vi "Dashboard Main.vi"() -> ()   [LabVIEW 2013]
uses:
  <vilib>/event_ctls.llb/eventvkey.ctl
  <vilib>/Rock Robotics/WPI/Dashboard/WPI_DashboardLogging Global.vi
  <vilib>/Utility/config.llb/Write Key (String).vi
  <vilib>/Utility/config.llb/Write Key (I32).vi
  <vilib>/Utility/config.llb/NI_LVConfig.lvlib
panel:
  out "Image Message":string="Timeout in Camera Communications"
  in  "Rec Mode":enum32{"Stop", "Record", "Playback"}(radio)
  in  "Dashboard Tab":T1(tab)
  out "Meter":dbl(knob) caption="Catapult Pressure" scale=0.0..100.0
  out "TapeMeasure":dbl caption="Distance To Target" format="%#_4g"
  out "CatapultLocked":bool caption="Catapult"
  out "TRghtStop":bool caption="Turret Right Stop"
  out "TLftStop":bool caption="Turret Left Stop"
  in  "Camera Settings":T2={"Frame Rate"=30, "Compression"=30, "Size"=1} {"Frame Rate" scale=1.0..30.0; "Size" items=["640x480", "320x240", "160x120"]}
  out "MotorSliders R":cluster{"MotorSlide1":dbl, "MotorSlide2":dbl} {"MotorSlide2" scale=-1.0..1.0 scale format="%#_2e"; "MotorSlide1" scale=-1.0..1.0 scale format="%#_2e"}
  out "MotorChart R":cluster{"Numeric":dbl, "Numeric":dbl}(graph)
  out "MotorSliders L":T3 {"MotorSlide4 2" scale=0.0..14.0 scale format="%#_2e"; "MotorSlide2" scale=-1.0..1.0 scale format="%#_2e"; "MotorSlide1" scale=-1.0..1.0 scale format="%#_2e"}
  out "MotorChart L":T4(graph)
  out "JS1 Z":dbl(slide) scale=-1.0..1.0 scale format="%#_2e"
  out "Joystick 1":cluster{"X":dbl, "Y":dbl}[](graph)
  out "JS Buttons 1":T5
  out "JS2 Z":dbl(slide) scale=-1.0..1.0 scale format="%#_2e"
  out "Joystick 2":cluster{"X":dbl, "Y":dbl}[](graph)
  out "JS Buttons 2":T5
  out "Mode":T6(ring)=enum."Auto Disabled"
  out "Camera IP":string
  in  "DB Camera Config":bool
  out "fps":dbl format="%#.1g"
  out "Mbps":dbl format="%#.1g"
  out "Mbps 2":bool
  out "JS3 Z":dbl(slide) scale=1.0..-1.0 scale format="%#_2e"
  out "Joystick 3":cluster{"X":dbl, "Y":dbl}[](graph) caption="XBOX"
  out "JS Buttons 3":T5
  in  "Slider 1":dbl(slide) scale=0.0..100.0
  in  "Checkbox 2":bool
  in  "Checkbox 1":bool
  in  "Test Slider":dbl(slide) scale=0.0..100.0 scale format="%#_3g"
  in  "On/Off":bool caption="Solenoid"
  in  "Test Name":u16(ring) items=["Select the test to run...", "Example Test", "-------------------------------", "List of tests is built in robot code.", "Replace with your own automated tests."]
  in  "Test Tree":string(tree)
  in  "Motor":cluster{"Value":dbl, "Enable":bool} {"Value" scale=-1.0..1.0 scale format="%#_3g"}
  out "Progress":T7 {"Test Progress" scale=0.0..100.0}
  in  "Rev/Fwd":cluster{"Forward":bool, "Reverse":bool}
  in  "Test Ring":u16(ring) items=["Auto", "Fixed indoor", "Fixed outdoor 1", "Fixed outdoor 2", "Fixed fluorescent 1", "Fixed fluorescent 2", "Hold current"]
  in  "Listbox":i32(listbox)
  out "Tree":string(tree)
  out "Camera Image":T8(plugin-control)
  in  "Enable":bool
  # "Left"
  # "Front"
  # "Right"
  # "Battery"
  # "Customize by placing controls and indicators here and name to\nmatch Dashboard Variables on robot."
  # "This tab is a great place for autonomous settings and validation.\nCustomize by placing controls and indicators here and name to\nmatch Dashboard Variables on robot."
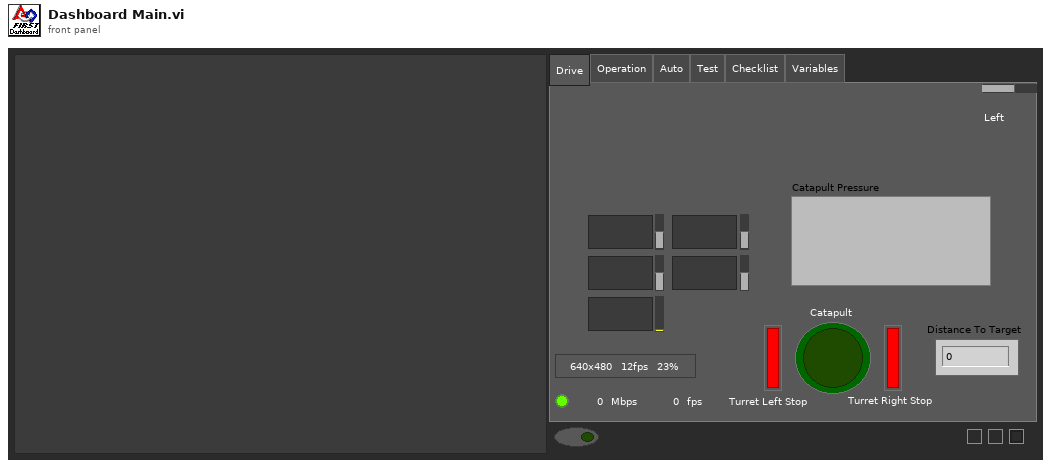
[diagram p1: front panel]
types:
  T1 = enum32{"Drive", "Operation", "Auto", "Test", "Checklist", "Variables"}
  T2 = cluster{"Frame Rate":i32, "Compression":i32, "Size":u16}
  T3 = cluster{"MotorSlide1":dbl, "MotorSlide2":dbl, "MotorSlide4 2":dbl}
  T4 = cluster{"Numeric":dbl, "Numeric":dbl, "Battery":sgl}
  T5 = cluster{bool, bool, bool, bool, bool, bool, bool, bool, bool, bool, bool, bool}
  T6 = enum8{"Tele-Op Disabled", "Tele-Op Enabled", "Auto Disabled", "Auto Enabled", "Test Disabled", "Test Enabled", ""}
  T7 = cluster{"Test Progress":u8, "Test Progress Text":string}
  T8 = typedef "IMAQ Image.ctl" = refnum<image>
  T9 = typedef "Image Type" = u32
  T10 = cluster{"Digital Inputs":bool[], "Digital Outputs":bool[]}
  T11 = cluster{"Competition mode":bool, "Robot Link":bool, "Autonomous":bool, "Enabled":bool, "E-Stop":bool, "Simulated":bool, "TestMode":bool, "Docked Window":bool}
  T12 = cluster{"Boolean Array[0]":bool, "Boolean Array[1]":bool, "Boolean Array[2]":bool, "Boolean Array[3]":bool, "Boolean Array[4]":bool, "Boolean Array[5]":bool, "Boolean Array[6]":bool, "Boolean Array[7]":bool, "Boolean Array[8]":bool, "Boolean Array[9]":bool, "Boolean Array[10]":bool, "Boolean Array[11]":bool}
  T13 = typedef "NI_LVConfig.lvlib/Config Data RefNum.ctl" = refnum<k1>
  T14 = typedef "eventvkey.ctl" = enum16{"ASCII", "Enter", "Return", "Shift", "Ctrl", "Alt", "Cmd", "Opt", "Caps", "NumLock", "Clear", "Break", "Up", "Down", "Left", "Right", "Insert", "Delete", "Home", "End", "PageUp", "PageDown", "Escape", "Help", "Pause", "ScrollLock", "F1", "F2", "F3", "F4", "F5", "F6", "F7", "F8", "F9", "F10", "F11", "F12", "F13", "F14", "F15", "F16", "F17", "F18", "F19", "F20", "F21", "F22", "F23", "F24", "Play", "VolumeUp", "VolumeDown", "Mute", "Two Byte Char"}
  T15 = cluster{"Image Size":bool, "Image Type":bool, "Pixel Value":bool, "ROI Information":bool, "Zoom Factor":bool}
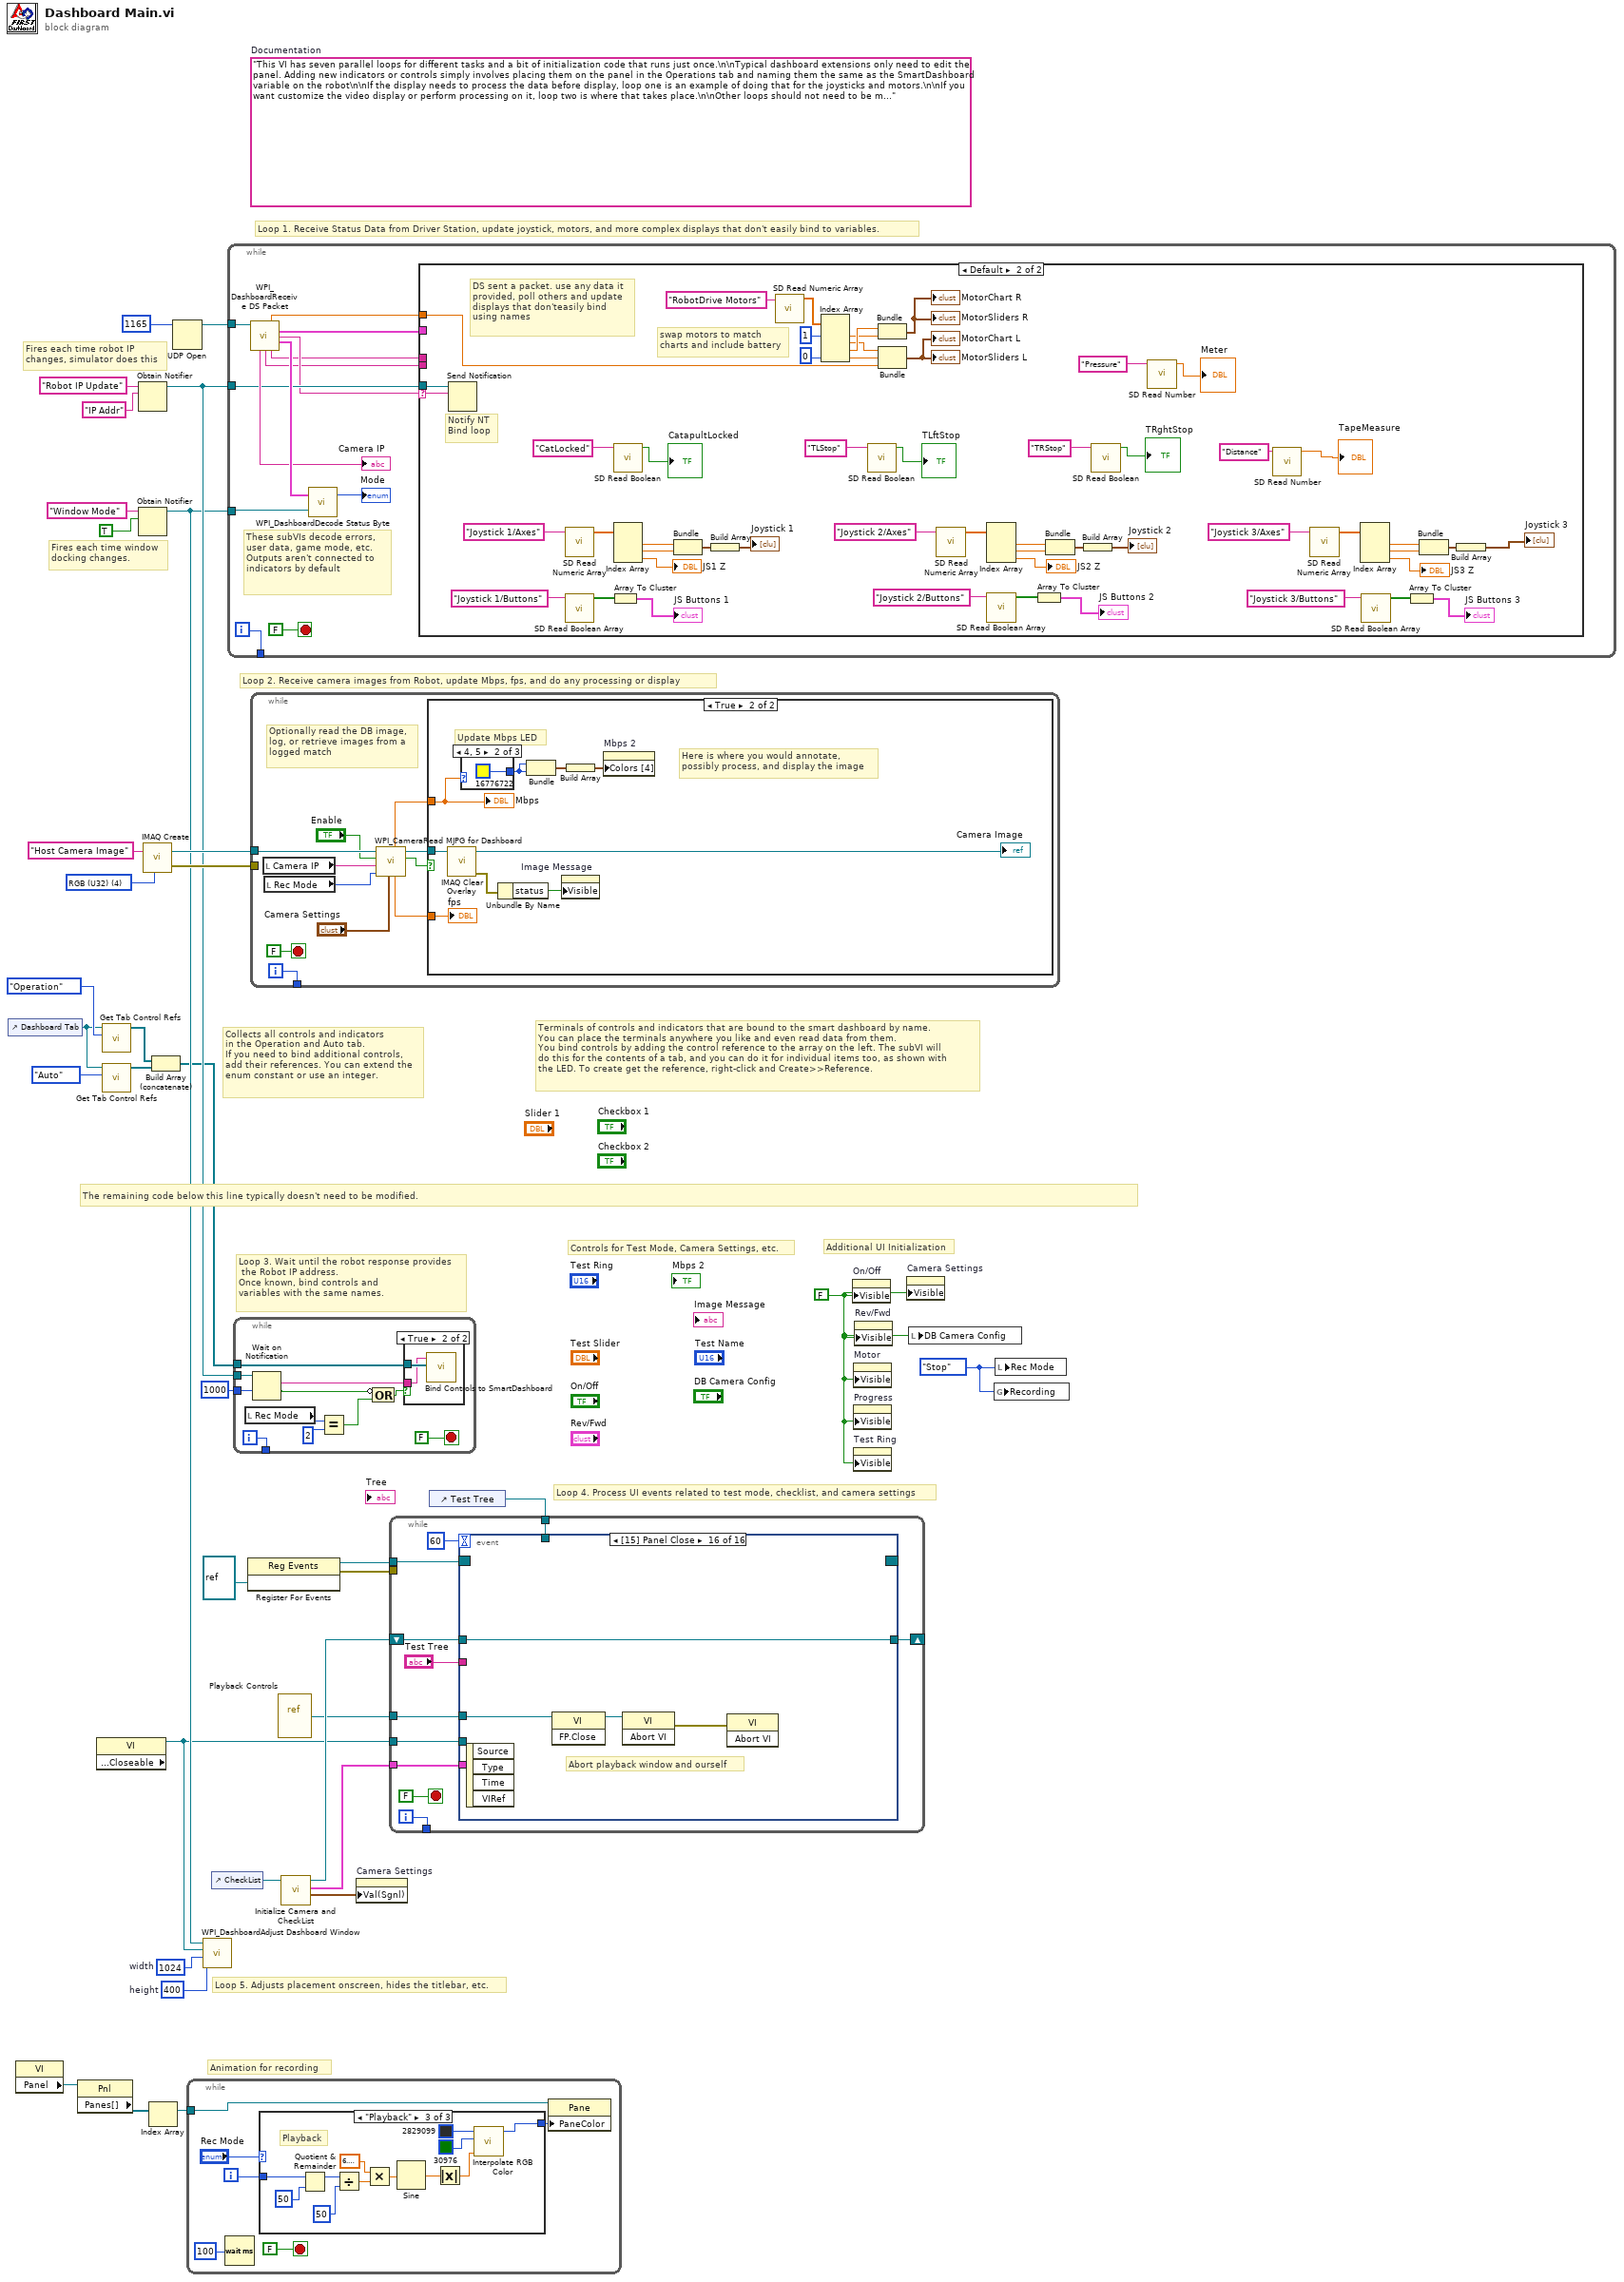
[diagram p0: block diagram]
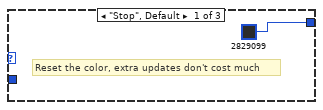
[diagram p2: hidden frame]
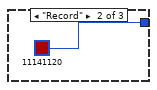
[diagram p3: hidden frame]
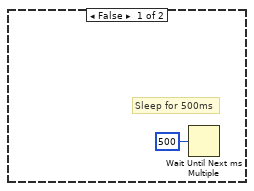
[diagram p5: hidden frame]
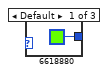
[diagram p6: hidden frame]
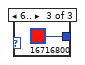
[diagram p7: hidden frame]
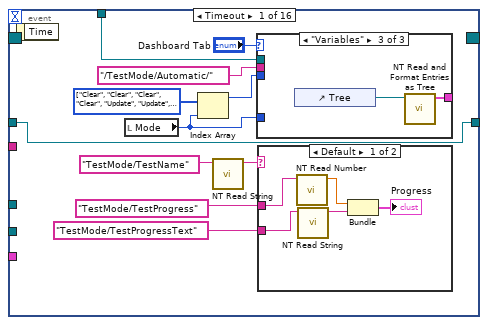
[diagram p8: hidden frame]
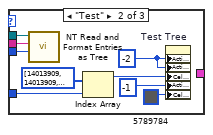
[diagram p10: hidden frame]
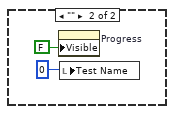
[diagram p11: hidden frame]
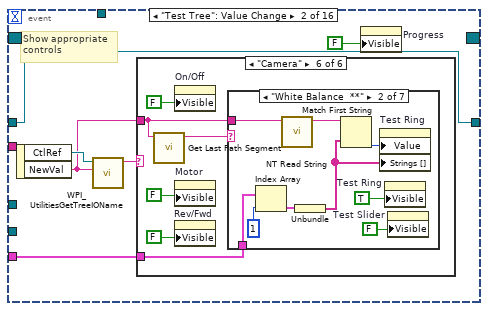
[diagram p12: hidden frame]
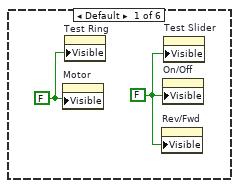
[diagram p13: hidden frame]
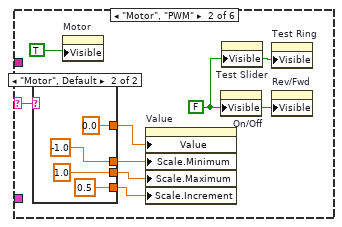
[diagram p14: hidden frame]
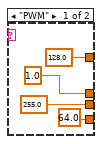
[diagram p15: hidden frame]
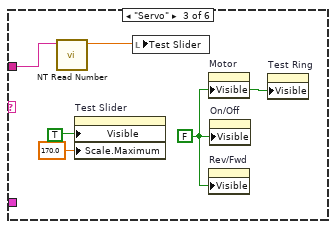
[diagram p16: hidden frame]
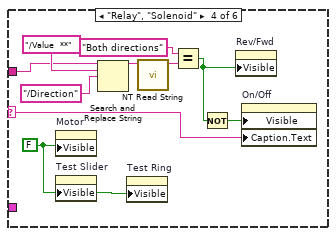
[diagram p17: hidden frame]
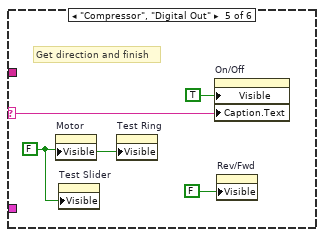
[diagram p18: hidden frame]
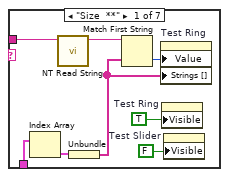
[diagram p19: hidden frame]
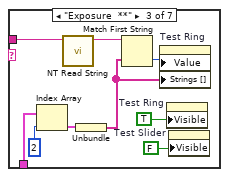
[diagram p20: hidden frame]
diagram:
  w7 = enum32{"Stop", "Record", "Playback"}."Stop" ("Rec Mode")
  w10 = 400  # height
  w11 = 1024  # width
  w24 = FALSE ("Visible")
  (unwired) "This VI has seven parallel loops for different tasks and a bit of initialization code that runs just once.\n\nTypical dashboard extensions only need to edit the panel. Adding new indicators or controls simply involves placing them on the panel in the Operations tab and naming them the same as the SmartDashboard variable on the robot\n\nIf the display needs to process the data before display, loop one is an example of doing that for the joysticks and motors.\n\nIf you want customize the video display or perform processing on it, loop two is where that takes place.\n\nOther loops should not need to be modified. They are pretty standard, and document the task they perform."  # Documentation
  w34 = T9 4 items=["Grayscale (U8)", "Grayscale (I16)", "Grayscale (SGL)", "Complex (CSG)", "RGB (U32)", "HSL (U32)", "RGB (U64)"] ("Image Type")
  # "Controls for Test Mode, Camera Settings, etc."
  # "Additional UI Initialization"
  # "Animation for recording"
  # "Fires each time robot IP\nchanges, simulator does this"
  # "Fires each time window\ndocking changes."
  # "Collects all controls and indicators\nin the Operation and Auto tab.\nIf you need to bind additional controls,\nadd their references. You can extend the\nenum constant or use an integer."
  # "The remaining code below this line typically doesn't need to be modified."
  # "Loop 4. Process UI events related to test mode, checklist, and camera settings"
  # "Terminals of controls and indicators that are bound to the smart dashboard by name.\nYou can place the terminals anywhere you like and even read data from them.\nYou bind controls by adding the control reference to the array on the left. The subVI will\ndo this for the contents of a tab, and you can do it for individual items too, as shown with\nthe LED. To create get the reference, right-click and Create>>Reference."
  # "Loop 3. Wait until the robot response provides\n the Robot IP address.\nOnce known, bind controls and\nvariables with the same names."
  # "Loop 5. Adjusts placement onscreen, hides the titlebar, etc."
  # "Loop 1. Receive Status Data from Driver Station, update joystick, motors, and more complex displays that don't easily bind to variables."
  # "Loop 2. Receive camera images from Robot, update Mbps, fps, and do any processing or display"
  n1 = control-ref of="Dashboard Tab"() -> (w5:refnum<vi>)
  n2 = property class="VI"() -> ("Panel"=w18:refnum<vi>)  [unwired: 2 in, 2 out]
  n3 = property class="Pnl"(reference=w18) -> ("Panes[]"=w19:refnum<vi>[])  [unwired: 1 in, 2 out]
  n4 = property class="VI" props=["Front Panel.Closeable"]() -> (reference out=w6:refnum<vi>)  [unwired: 2 in, 2 out]
  n5 = call <vilib>:"Get Tab Control Refs.vi"("Page Index"=T1."Operation" ("Dashboard Tab"), "TabControl in"=w5) -> ("ControlsOnPage"=w3:refnum<vi>[])  [unwired: 9 in]
  n6 = call <vilib>:"Get Tab Control Refs.vi"("Page Index"=T1."Auto" ("Dashboard Tab"), "TabControl in"=w5) -> ("ControlsOnPage"=w4:refnum<vi>[])  [unwired: 9 in]
  n7 = Obtain Notifier(name (unnamed)="Robot IP Update", notification data type="IP Addr" ("name (unnamed)")) -> (notifier out=w28:refnum<notifier>)  [unwired: 2 in, 2 out]
  n8 = Obtain Notifier(name (unnamed)="Window Mode", notification data type=TRUE) -> (notifier out=w9:refnum<notifier>)  [unwired: 2 in, 2 out]
  n9 = call "IMAQ Create"("Image Name"="Host Camera Image", "Image Type"=w34) -> ("New Image"=w32:T8, "error out"=w31:errorcluster)  [unwired: 2 in, 1 out]
  n10 = Index Array(array=w19) -> (element=w17:refnum<vi>)  [unwired: 1 in]
  n11 = Build Array (concatenate)(w3, w4) -> (w2:refnum<vi>[])
  n12 = UDP Open(11:u16 1165 ("port")) -> (port=w35:refnum<k16>)  [unwired: 2 in, 4 out]
  n13 = while {
    tunnel: w17 -> [w38]
    i -> [w41]
    stop <- FALSE stop-if-true
    n14 = Wait (ms)(milliseconds to wait=u32 100) -> ()  [unwired: 1 out]
    n15 = case shown="\"Playback\"" "Rec Mode" {
      tunnel: w41 -> [_ _ w56]
      tunnel: [u32 2829099 ("Base Color") u32 11141120 ("Target Color") w45] -> w37
      frame "Stop", Default {
        # "Reset the color, extra updates don't cost much"
      }
      frame "Record" {
      }
      frame "Playback" {
        # "Playback"
        n16 = Quotient & Remainder(x=w56, y=u32 50 ("milliseconds to wait")) -> (x-y*floor(x/y)=w52:u32)  [unwired: 1 out]
        n17 = Divide(x=w52, y=u32 50 ("milliseconds to wait")) -> (x/y=w49:dbl)
        n18 = Multiply(x=6.283185307179586, y=w49) -> (x*y=w54:dbl)
        n19 = Sine(x=w54) -> (sin(x)=w53:dbl)
        n20 = Absolute Value(x=w53) -> (abs(x)=w46:dbl)
        n21 = call "Interpolate RGB Color.vi"("Proportion"=w46, "Target Color"=u32 30976, "Base Color"=u32 2829099) -> ("Result Color"=w45:u32)  [unwired: 8 in]
      }
    }
    n22 = property class="Pane"(reference=w38, "PaneColor"=w37) -> ()  [unwired: 1 in, 2 out]
  }
  n23 = call <vilib>:"WPI_DashboardAdjust Dashboard Window.vi"("height"=w10, "width"=w11, "reference in"=w6, "Notifier in"=w9) -> ()  [unwired: 8 in]
  n24 = control-ref of="CheckList"() -> (w8:refnum<vi>)
  n25 = while {
    tunnel: w35 -> [w67]
    tunnel: w28 -> [w62]
    tunnel: w9 -> [w66]
    tunnel: [w63] -> _
    i -> [w63]
    stop <- FALSE stop-if-true
    # "These subVIs decode errors, user data, game mode, etc.\nOutputs aren't connected to indicators by default"
    n26 = call <vilib>:"WPI_DashboardReceive DS Packet.vi"("Recv Socket"=w67) -> ("Battery"=w57:sgl, "Driver Station"=w58:T10, "Robot IP Address"=w61:string, "Status"=w68:T11, "Camera IP Address"=→"Camera IP":string, "Low Priority User Data"=w60:string, "High Priority User Data"=w59:string)  [unwired: 1 in, 7 out]
    n27 = call <vilib>:"WPI_DashboardDecode Status Byte.vi"("Window Mode Notifier"=w66, "Status"=w68) -> ("Mode"=→"Mode":T6)  [unwired: 1 out]
    n28 = case shown="Default" w61 {
      selector: w61 -> [_ w100]
      tunnel: w62 -> [_ w101]
      tunnel: w60 -> [_ _]
      tunnel: w59 -> [_ _]
      tunnel: w58 -> [_ _]
      tunnel: w57 -> [_ w99]
      frame "0.0.0.0" {
        # "DS not sending packets, or no robot exists yet.\nDon't poll the variables"
      }
      frame Default {
        # "Notify NT\nBind loop"
        # "DS sent a packet. use any data it\nprovided, poll others and update\ndisplays that don'teasily bind\nusing names"
        # "swap motors to match\ncharts and include battery"
        n29 = Send Notification(notification=w100, notifier=w101) -> ()  [unwired: 1 in, 2 out]
        n30 = call <vilib>:"SD Read Numeric Array.vi"("Name"="Joystick 1/Axes") -> ("Numeric Array"=w117:dbl[])  [unwired: 8 in, 2 out]
        n31 = call <vilib>:"SD Read Boolean Array.vi"("Name"="Joystick 1/Buttons") -> ("Boolean Array"=w119:bool[])  [unwired: 8 in, 2 out]
        n32 = Array To Cluster(array=w119) -> (cluster=→"JS Buttons 1":T12)
        n33 = call <vilib>:"SD Read Boolean.vi"("Name"="CatLocked") -> ("Boolean"=→"CatapultLocked":bool)  [unwired: 8 in, 2 out]
        n34 = Index Array(array=w117) -> (element #1=w114:dbl, element #2=w115:dbl, element #3=→"JS1 Z":dbl)  [unwired: 3 in]
        n35 = Bundle("Numeric"=w114, "Numeric"=w115) -> (w113:cluster{"Numeric":dbl, "Numeric":dbl})  [unwired: 1 in]
        n36 = Build Array(w113) -> (→"Joystick 1":cluster{"Numeric":dbl, "Numeric":dbl}[])
        n37 = call <vilib>:"SD Read Numeric Array.vi"("Name"="RobotDrive Motors") -> ("Numeric Array"=w98:dbl[])  [unwired: 8 in, 2 out]
        n38 = Index Array(array=w98, index #1=1, index #4=0) -> (element #1=w94:dbl, element #2=w93:dbl, element #3=w95:dbl, element #4=w90:dbl)  [unwired: 2 in]
        n39 = call <vilib>:"SD Read Boolean.vi"("Name"="TLStop") -> ("Boolean"=→"TLftStop":bool)  [unwired: 8 in, 2 out]
        n40 = Bundle("Numeric"=w95, "Numeric"=w94) -> (→"MotorChart R" →"MotorSliders R":cluster{"Numeric":dbl, "Numeric":dbl})  [unwired: 1 in]
        n41 = Bundle("Numeric"=w93, "Numeric"=w90, "Battery"=w99) -> (→"MotorChart L" →"MotorSliders L":T4)  [unwired: 1 in]
        n42 = call <vilib>:"SD Read Numeric Array.vi"("Name"="Joystick 2/Axes") -> ("Numeric Array"=w111:dbl[])  [unwired: 8 in, 2 out]
        n43 = Index Array(array=w111) -> (element #1=w106:dbl, element #2=w105:dbl, element #3=→"JS2 Z":dbl)  [unwired: 3 in]
        n44 = call <vilib>:"SD Read Boolean Array.vi"("Name"="Joystick 2/Buttons") -> ("Boolean Array"=w110:bool[])  [unwired: 8 in, 2 out]
        n45 = Array To Cluster(array=w110) -> (cluster=→"JS Buttons 2":T12)
        n46 = Bundle("Numeric"=w106, "Numeric"=w105) -> (w107:cluster{"Numeric":dbl, "Numeric":dbl})  [unwired: 1 in]
        n47 = Build Array(w107) -> (→"Joystick 2":cluster{"Numeric":dbl, "Numeric":dbl}[])
        n48 = call <vilib>:"SD Read Boolean.vi"("Name"="TRStop") -> ("Boolean"=→"TRghtStop":bool)  [unwired: 8 in, 2 out]
        n49 = call <vilib>:"SD Read Number.vi"("Name"="Pressure") -> ("Numeric"=→"Meter":dbl)  [unwired: 8 in, 2 out]
        n50 = call <vilib>:"SD Read Number.vi"("Name"="Distance") -> ("Numeric"=→"TapeMeasure":dbl)  [unwired: 8 in, 2 out]
        n51 = call <vilib>:"SD Read Numeric Array.vi"("Name"="Joystick 3/Axes") -> ("Numeric Array"=w80:dbl[])  [unwired: 8 in, 2 out]
        n52 = Index Array(array=w80) -> (element #1=w77:dbl, element #2=w76:dbl, element #3=→"JS3 Z":dbl)  [unwired: 3 in]
        n53 = call <vilib>:"SD Read Boolean Array.vi"("Name"="Joystick 3/Buttons") -> ("Boolean Array"=w83:bool[])  [unwired: 8 in, 2 out]
        n54 = Array To Cluster(array=w83) -> (cluster=→"JS Buttons 3":T12)
        n55 = Bundle("Numeric"=w77, "Numeric"=w76) -> (w78:cluster{"Numeric":dbl, "Numeric":dbl})  [unwired: 1 in]
        n56 = Build Array(w78) -> (→"Joystick 3":cluster{"Numeric":dbl, "Numeric":dbl}[])
      }
    }
  }
  n57 = while {
    tunnel: w2 -> [w133]
    tunnel: w28 -> [w131]
    tunnel: [w129] -> _
    tunnel: u32 1000 ("milliseconds to wait") -> [w128]
    i -> [w129]
    stop <- FALSE stop-if-true
    n58 = local read "Rec Mode"() -> (w124:enum32{"Stop", "Record", "Playback"})
    n59 = Wait on Notification(notifier=w131, timeout in ms (-1)=w128) -> (notification=w130:string, timed out?=w126:bool)  [unwired: 2 in, 2 out]
    n60 = Equal?(x=w124, y=u16 2 ("Rec Mode")) -> (x = y?=w125:bool)
    n61 = Compound Arithmetic op=OR(invert w126, w125) -> (w127:bool)
    n62 = case shown="True" w127 {
      tunnel: w133 -> [_ w135]
      tunnel: w130 -> [_ w134]
      frame False {
      }
      frame True {
        n63 = call <vilib>:"Bind Controls to SmartDashboard.vi"("Bound Control Refs"=w135, "Server IP Address"=w134) -> ()  [unwired: 10 in]
      }
    }
  }
  n64 = register-events(refnum<vi> refnum) -> (reference out=w15:refnum<event-registration>, error out=w14:errorcluster)  [unwired: 2 in]
  n65 = while {
    tunnel: w32 -> [w144]
    tunnel: w31 -> [_]
    tunnel: [w145] -> _
    i -> [w145]
    stop <- FALSE stop-if-true
    # "Optionally read the DB image,\nlog, or retrieve images from a\nlogged match"
    n66 = local read "Camera IP"() -> (w137:string)
    n67 = local read "Rec Mode"() -> (w136:enum32{"Stop", "Record", "Playback"})
    n68 = call <vilib>:"WPI_CameraRead MJPG for Dashboard.vi"("Camera Settings"="Camera Settings", "Rec Mode"=w136, "Camera IP"=w137, "Enable"="Enable", "Refnum in"=w144) -> ("Active"=w141:bool, "Refnum out"=w143:T8, "FPS"=w140:dbl, "Bandwidth (Mbps)"=w139:dbl)  [unwired: 3 in]
    n69 = case shown="True" w141 {
      tunnel: w143 -> [_ w151]
      tunnel: w139 -> [_ w150]
      tunnel: w140 -> [_ w148]
      frame False {
        # "Sleep for 500ms"
        n70 = Wait Until Next ms Multiple(millisecond multiple=u32 500) -> ()  [unwired: 1 out]
      }
      frame True {
        # "Here is where you would annotate,\npossibly process, and display the image"
        # "Update Mbps LED"
        n71 = call "IMAQ Clear Overlay"("Image"=w151) -> ("error out"=w155:errorcluster, "Image Out"=→"Camera Image":T8)  [unwired: 2 in, 7 out]
        n72 = case shown="4, 5" w150 {
          tunnel: [u32 6618880 ("Color Box") u32 16776722 ("Color Box") u32 16716800 ("Color Box")] -> w152
          frame Default {
          }
          frame 4, 5 {
          }
          frame 6.. {
          }
        }
        n73 = Unbundle By Name(w155) -> ("status"=w156:bool)
        n74 = Bundle("Color Box"=w152, "Color Box"=w152) -> (w154:cluster{"Color Box":u32, "Color Box":u32})  [unwired: 1 out]
        n75 = property on="Image Message" class="Str"("Visible"=w156) -> ()  [unwired: 2 in, 2 out]
        n76 = Build Array(w154) -> (w153:cluster{"Color Box":u32, "Color Box":u32}[])
        n77 = property on="Mbps 2" class="Bool (strict)"("Colors [4]"=w153) -> ()  [unwired: 2 in, 2 out]
        "Mbps" <- w150
        "fps" <- w148
      }
    }
  }
  n78 = vi-ref "Playback Controls.vi"() -> (w16:refnum<vi>)
  n79 = call "Initialize Camera and CheckList.vi"("ListBox in"=w8) -> ("Cluster"=w22:cluster{"value":i32, "value":i32, "index":i32}, "Array"=w23:cluster{string[]}[], "File Refnum"=w21:T13)  [unwired: 8 in]
  n80 = property on="Camera Settings" class="Clust (strict)"("Val(Sgnl)"=w22) -> ()  [unwired: 2 in, 2 out]
  n81 = control-ref of="Test Tree"() -> (w20:refnum<vi>)
  n82 = while {
    tunnel: w23 -> [w167]
    shift-right: [w166] -> _
    shift-left: w21 -> [w165]
    tunnel: [w164] -> _
    tunnel: w20 -> [w163]
    tunnel: w16 -> [w162]
    tunnel: w15 -> [w161]
    tunnel: w14 -> [_]
    tunnel: w6 -> [w160]
    i -> [w164]
    stop <- FALSE stop-if-true
    n83 = event shown="[15] Panel Close" {
      selector: w161 -> [_ _ _ _ _ _ _ _ _ _ _ _ _ _ _ _]
      dyn-events: [_ _ _ _ _ _ _ _ _ _ _ _ _ w405 _ _] -> _
      timeout: u32 60 ("milliseconds to wait") -> [_ _ _ _ _ _ _ _ _ _ _ _ _ _ _ _]
      tunnel: w163 -> [w177 _ _ _ _ _ _ _ _ _ _ _ _ _ _ _]
      tunnel: "Test Tree" -> [_ _ _ _ _ _ _ _ w374 w382 w384 w388 w396 _ _ _]
      tunnel: w167 -> [_ w201 _ _ _ _ w338 w368 _ _ _ _ _ _ _ _]
      tunnel: [w171 w200 w299 w304 w312 w324 w337 w361 w373 w380 w383 w387 w395 w407 w421 w422] -> w166
      tunnel: w165 -> [w171 w200 w299 w304 w312 w324 w336 w361 w373 w380 w383 w387 w395 w407 w421 w422]
      tunnel: w162 -> [_ _ _ _ _ _ _ _ _ _ _ _ _ w408 _ w425]
      tunnel: w160 -> [_ _ _ _ _ _ _ _ _ _ _ _ _ w403 _ _]
      event Timeout {
        w176 = enum16{"Update", "Clear"}[] [enum."Clear", enum."Clear", enum."Clear", enum."Clear", enum."Update", enum."Update", enum."Clear"] items=["Update", "Clear"]
        n84 = event-data() -> ()  [unwired: 1 in, 1 out]
        n85 = local read "Mode"() -> (w174:T6)
        n86 = Index Array(array=w176, index=w174) -> (element=w175:enum16{"Update", "Clear"})
        n87 = call <vilib>:"NT Read String.vi"("Name"="TestMode/TestName") -> ("String"=w180:string)  [unwired: 9 in, 1 out]
        n88 = case shown="\"Variables\"" "Dashboard Tab" {
          tunnel: w177 -> [_ w190 _]
          tunnel: "/TestMode/Automatic/" ("Name Pattern") -> [_ w189 _]
          tunnel: w175 -> [_ w188 _]
          tunnel: w174 -> [_ w186 _]
          tunnel: [_ _ w192] -> _
          frame "Operation", Default {
          }
          frame "Test" {
            w185 = -2 ("Active Item:Row Number")
            n89 = call <vilib>:"NT Read and Format Entries as Tree.vi"("Operation"=w188, "Name Pattern"=w189, "Tree Refnum"=w190) -> ()  [unwired: 7 in, 2 out]
            n90 = Index Array(array=u32[] [14013909, 14013909, 14013909, 14013909, 14013909, 16777215, 14013909], index=w186) -> (element=w184:u32)
            n91 = property on="Test Tree" class="Tree (strict)"("Active Item Row Number"=w185, "ActiveColNum"=w185, "CellBG"=w184, "Active Item Row Number"=-1 ("Active Item:Row Number"), "CellBG"=u32 5789784 ("Color Box")) -> ()  [unwired: 2 in, 2 out]
          }
          frame "Variables" {
            n92 = control-ref of="Tree"() -> (w191:refnum<vi>)
            n93 = call <vilib>:"NT Read and Format Entries as Tree.vi"("Tree Refnum"=w191) -> ("Formatted Strings"=w192:cluster{"Name":string, "Value":string}[])  [unwired: 9 in, 1 out]
          }
        }
        n94 = case shown="Default" w180 {
          tunnel: "TestMode/TestProgress" ("Name") -> [w194 _]
          tunnel: "TestMode/TestProgressText" ("Name") -> [w193 _]
          frame Default {
            n95 = call <vilib>:"NT Read Number.vi"("Name"=w194) -> ("Numeric"=w195:dbl)  [unwired: 9 in, 1 out]
            n96 = call <vilib>:"NT Read String.vi"("Name"=w193) -> ("String"=w196:string)  [unwired: 9 in, 1 out]
            n97 = Bundle("Numeric"=w195, "String"=w196) -> (→"Progress":cluster{"Numeric":dbl, "String":string})  [unwired: 1 in]
          }
          frame "" {
            n98 = property on="Progress" class="Clust (strict)"("Visible"=FALSE) -> ()  [unwired: 2 in, 2 out]
            n99 = local write "Test Name"(u16 0) -> ()
          }
        }
      }
      event "Test Tree": Value Change {
        # "Show appropriate\ncontrols"
        n100 = event-data() -> ("CtlRef"=w204:refnum<vi>, "NewVal"=w202:string)  [unwired: 1 in]
        n101 = call <vilib>:"WPI_UtilitiesGetTreeIOName.vi"("NewVal"=w202, "TreeControl in"=w204) -> ("I/O Name"=w205:string)  [unwired: 9 in]
        n102 = case shown="\"Camera\"" w205 {
          selector: w205 -> [_ w212 _ w230 w239 _]
          tunnel: w202 -> [_ _ w227 w229 _ w246]
          tunnel: w201 -> [_ _ _ _ _ w245]
          frame Default {
            w207 = FALSE ("Visible")
            w206 = FALSE ("Visible")
            n103 = property on="Motor" class="Clust (strict)"("Visible"=w206) -> ()  [unwired: 2 in, 2 out]
            n104 = property on="Test Ring" class="Ring (strict)"("Visible"=w206) -> ()  [unwired: 2 in, 2 out]
            n105 = property on="Rev/Fwd" class="Clust (strict)"("Visible"=w207) -> ()  [unwired: 2 in, 2 out]
            n106 = property on="On/Off" class="Bool (strict)"("Visible"=w207) -> ()  [unwired: 2 in, 2 out]
            n107 = property on="Test Slider" class="Slide (strict)"("Visible"=w207) -> ()  [unwired: 2 in, 2 out]
          }
          frame "Motor", "PWM" {
            w213 = FALSE ("Visible")
            n108 = case shown="\"Motor\", Default" w212 {
              tunnel: [1.0 ("Value") -1.0 ("Value")] -> w211
              tunnel: [255.0 ("Value") 1.0 ("Value")] -> w210
              tunnel: [128.0 ("Value") 0.0 ("Value")] -> w209
              tunnel: [64.0 ("Value") 0.5 ("Value")] -> w208
              frame "PWM" {
              }
              frame "Motor", Default {
              }
            }
            n109 = property on="Motor" class="Clust (strict)"("Visible"=TRUE) -> ()  [unwired: 2 in, 2 out]
            n110 = property on="Value" class="Slide (strict)"("Value"=w209, "Scale.Minimum"=w211, "Scale.Maximum"=w210, "Scale.Increment"=w208) -> ()  [unwired: 2 in, 2 out]
            n111 = property on="On/Off" class="Bool (strict)"("Visible"=w213) -> ()  [unwired: 2 in, 2 out]
            n112 = property on="Test Slider" class="Slide (strict)"("Visible"=w213) -> ()  [unwired: 2 in, 2 out]
            n113 = property on="Test Ring" class="Ring (strict)"("Visible"=w213) -> ()  [unwired: 2 in, 2 out]
            n114 = property on="Rev/Fwd" class="Clust (strict)"("Visible"=w213) -> ()  [unwired: 2 in, 2 out]
          }
          frame "Servo" {
            w225 = FALSE ("Visible")
            n115 = call <vilib>:"NT Read Number.vi"("Name"=w227) -> ("Numeric"=w226:dbl)  [unwired: 9 in, 1 out]
            n116 = property on="Test Slider" class="Slide (strict)"("Visible"=TRUE, "Scale.Maximum"=170.0 ("Scale.Range:Maximum")) -> ()  [unwired: 2 in, 2 out]
            n117 = local write "Test Slider"(w226) -> ()
            n118 = property on="Motor" class="Clust (strict)"("Visible"=w225) -> ()  [unwired: 2 in, 2 out]
            n119 = property on="Rev/Fwd" class="Clust (strict)"("Visible"=w225) -> ()  [unwired: 2 in, 2 out]
            n120 = property on="On/Off" class="Bool (strict)"("Visible"=w225) -> ()  [unwired: 2 in, 2 out]
            n121 = property on="Test Ring" class="Ring (strict)"("Visible"=w225) -> ()  [unwired: 2 in, 2 out]
          }
          frame "Relay", "Solenoid" {
            w228 = FALSE ("Visible")
            n122 = property on="Motor" class="Clust (strict)"("Visible"=w228) -> ()  [unwired: 2 in, 2 out]
            n123 = property on="Test Slider" class="Slide (strict)"("Visible"=w228) -> ()  [unwired: 2 in, 2 out]
            n124 = Search and Replace String(input string=w229, search string="/Value  **", replace string="/Direction") -> (result string=w235:string)  [unwired: 5 in, 3 out]
            n125 = property on="Test Ring" class="Ring (strict)"("Visible"=w228) -> ()  [unwired: 2 in, 2 out]
            n126 = call <vilib>:"NT Read String.vi"("Name"=w235) -> ("String"=w233:string)  [unwired: 9 in, 1 out]
            n127 = Equal?(x="Both directions", y=w233) -> (x = y?=w231:bool)
            n128 = Not(x=w231) -> (.not. x?=w232:bool)
            n129 = property on="Rev/Fwd" class="Clust (strict)"("Visible"=w231) -> ()  [unwired: 2 in, 2 out]
            n130 = property on="On/Off" class="Bool (strict)"("Visible"=w232, "Caption.Text"=w230) -> ()  [unwired: 2 in, 2 out]
          }
          frame "Compressor", "Digital Out" {
            w238 = FALSE ("Visible")
            # "Get direction and finish"
            n131 = property on="Motor" class="Clust (strict)"("Visible"=w238) -> ()  [unwired: 2 in, 2 out]
            n132 = property on="Test Slider" class="Slide (strict)"("Visible"=w238) -> ()  [unwired: 2 in, 2 out]
            n133 = property on="Test Ring" class="Ring (strict)"("Visible"=w238) -> ()  [unwired: 2 in, 2 out]
            n134 = property on="On/Off" class="Bool (strict)"("Visible"=TRUE, "Caption.Text"=w239) -> ()  [unwired: 2 in, 2 out]
            n135 = property on="Rev/Fwd" class="Clust (strict)"("Visible"=FALSE) -> ()  [unwired: 2 in, 2 out]
          }
          frame "Camera" {
            n136 = call <vilib>:"Get Last Path Segment.vi"("String in"=w246) -> ("String out"=w247:string)  [unwired: 10 in]
            n137 = property on="On/Off" class="Bool (strict)"("Visible"=FALSE) -> ()  [unwired: 2 in, 2 out]
            n138 = property on="Motor" class="Clust (strict)"("Visible"=FALSE) -> ()  [unwired: 2 in, 2 out]
            n139 = property on="Rev/Fwd" class="Clust (strict)"("Visible"=FALSE) -> ()  [unwired: 2 in, 2 out]
            n140 = case shown="\"White Balance  **\"" w247 {
              tunnel: w246 -> [w253 w262 w271 w280 w289 _ w295]
              tunnel: w245 -> [w251 w259 w268 w277 w286 _ _]
              frame "Size  **" {
                n141 = Index Array(array=w251) -> (element=w250:cluster{string[]})  [unwired: 1 in]
                n142 = call <vilib>:"NT Read String.vi"("Name"=w253) -> ("String"=w252:string)  [unwired: 9 in, 1 out]
                n143 = Unbundle(w250) -> (w248:string[])
                n144 = Match First String(2:w248, 3:w252) -> (0:w249:i32)  [unwired: 1 out]
                n145 = property on="Test Ring" class="Ring (strict)"("Value"=w249, "Strings []"=w248) -> ()  [unwired: 2 in, 2 out]
                n146 = property on="Test Ring" class="Ring (strict)"("Visible"=TRUE) -> ()  [unwired: 2 in, 2 out]
                n147 = property on="Test Slider" class="Slide (strict)"("Visible"=FALSE) -> ()  [unwired: 2 in, 2 out]
              }
              frame "White Balance  **" {
                n148 = Index Array(array=w259, index=1) -> (element=w260:cluster{string[]})
                n149 = call <vilib>:"NT Read String.vi"("Name"=w262) -> ("String"=w261:string)  [unwired: 9 in, 1 out]
                n150 = Unbundle(w260) -> (w257:string[])
                n151 = Match First String(2:w257, 3:w261) -> (0:w256:i32)  [unwired: 1 out]
                n152 = property on="Test Ring" class="Ring (strict)"("Value"=w256, "Strings []"=w257) -> ()  [unwired: 2 in, 2 out]
                n153 = property on="Test Ring" class="Ring (strict)"("Visible"=TRUE) -> ()  [unwired: 2 in, 2 out]
                n154 = property on="Test Slider" class="Slide (strict)"("Visible"=FALSE) -> ()  [unwired: 2 in, 2 out]
              }
              frame "Exposure  **" {
                n155 = Index Array(array=w268, index=2) -> (element=w269:cluster{string[]})
                n156 = call <vilib>:"NT Read String.vi"("Name"=w271) -> ("String"=w270:string)  [unwired: 9 in, 1 out]
                n157 = Unbundle(w269) -> (w265:string[])
                n158 = Match First String(2:w265, 3:w270) -> (0:w266:i32)  [unwired: 1 out]
                n159 = property on="Test Ring" class="Ring (strict)"("Value"=w266, "Strings []"=w265) -> ()  [unwired: 2 in, 2 out]
                n160 = property on="Test Ring" class="Ring (strict)"("Visible"=TRUE) -> ()  [unwired: 2 in, 2 out]
                n161 = property on="Test Slider" class="Slide (strict)"("Visible"=FALSE) -> ()  [unwired: 2 in, 2 out]
              }
              frame "Exposure Priority  **" {
                n162 = Index Array(array=w277, index=3) -> (element=w278:cluster{string[]})
                n163 = call <vilib>:"NT Read String.vi"("Name"=w280) -> ("String"=w279:string)  [unwired: 9 in, 1 out]
                n164 = Unbundle(w278) -> (w274:string[])
                n165 = Match First String(2:w274, 3:w279) -> (0:w275:i32)  [unwired: 1 out]
                n166 = property on="Test Ring" class="Ring (strict)"("Value"=w275, "Strings []"=w274) -> ()  [unwired: 2 in, 2 out]
                n167 = property on="Test Ring" class="Ring (strict)"("Visible"=TRUE) -> ()  [unwired: 2 in, 2 out]
                n168 = property on="Test Slider" class="Slide (strict)"("Visible"=FALSE) -> ()  [unwired: 2 in, 2 out]
              }
              frame "Color Enable  **" {
                n169 = Index Array(array=w286, index=4) -> (element=w287:cluster{string[]})
                n170 = call <vilib>:"NT Read String.vi"("Name"=w289) -> ("String"=w288:string)  [unwired: 9 in, 1 out]
                n171 = Unbundle(w287) -> (w283:string[])
                n172 = Match First String(2:w283, 3:w288) -> (0:w284:i32)  [unwired: 1 out]
                n173 = property on="Test Ring" class="Ring (strict)"("Value"=w284, "Strings []"=w283) -> ()  [unwired: 2 in, 2 out]
                n174 = property on="Test Ring" class="Ring (strict)"("Visible"=TRUE) -> ()  [unwired: 2 in, 2 out]
                n175 = property on="Test Slider" class="Slide (strict)"("Visible"=FALSE) -> ()  [unwired: 2 in, 2 out]
              }
              frame Default {
                n176 = property on="Test Ring" class="Ring (strict)"("Visible"=FALSE) -> ()  [unwired: 2 in, 2 out]
                n177 = property on="Test Slider" class="Slide (strict)"("Visible"=FALSE) -> ()  [unwired: 2 in, 2 out]
              }
              frame "Brightness  **", "Color Level  **", "Compression  **", "FPS  **", "Sharpness  **" {
                n178 = call <vilib>:"NT Read Number.vi"("Name"=w295) -> ("Numeric"=w294:dbl)  [unwired: 9 in, 1 out]
                n179 = local write "Test Slider"(w294) -> ()
                n180 = property on="Test Slider" class="Slide (strict)"("Visible"=TRUE, "Scale.Maximum"=100.0 ("Scale.Range:Maximum")) -> ()  [unwired: 2 in, 2 out]
                n181 = property on="Test Ring" class="Ring (strict)"("Visible"=FALSE) -> ()  [unwired: 2 in, 2 out]
              }
            }
          }
        }
        n182 = property on="Progress" class="Clust (strict)"("Visible"=FALSE) -> ()  [unwired: 2 in, 2 out]
      }
      event "Test Name": Mouse Enter {
        # "Populate the ring with the list of tests"
        n183 = event-data() -> ()  [unwired: 1 in, 1 out]
        n184 = call <vilib>:"NT Read String Array.vi"("Name"="TestMode/TestList") -> ("String Array"=w303:string[])  [unwired: 9 in, 1 out]
        n185 = Build Array (concatenate)("Select the test to run...", w303) -> (w302:string[])
        n186 = property on="Test Name" class="Ring (strict)"("Strings []"=w302) -> ()  [unwired: 2 in, 2 out]
      }
      event "Test Name": Value Change {
        w305 = FALSE ("Visible")
        # "Tell the robot the test name to run"
        n187 = event-data() -> ("NewVal"=w309:u16)  [unwired: 1 in]
        n188 = property on="Test Name" class="Ring (strict)"() -> ("Strings []"=w310:string[])  [unwired: 2 in, 2 out]
        n189 = local write "Progress"(T7 {"Test Progress"=0, "Test Progress Text"=""} ("Progress")) -> ()
        n190 = Index Array(array=w310, index=w309) -> (element=w308:string)
        n191 = call <vilib>:"NT Write String.vi"("String"=w308, "Name"="TestMode/TestName") -> ()  [unwired: 9 in, 1 out]
        n192 = property on="Progress" class="Clust (strict)"("Visible"=TRUE) -> ()  [unwired: 2 in, 2 out]
        n193 = property on="Motor" class="Clust (strict)"("Visible"=w305) -> ()  [unwired: 2 in, 2 out]
        n194 = property on="Test Slider" class="Slide (strict)"("Visible"=w305) -> ()  [unwired: 2 in, 2 out]
        n195 = property on="On/Off" class="Bool (strict)"("Visible"=w305) -> ()  [unwired: 2 in, 2 out]
        n196 = property on="Rev/Fwd" class="Clust (strict)"("Visible"=w305) -> ()  [unwired: 2 in, 2 out]
        n197 = property on="Test Ring" class="Ring (strict)"("Visible"=w305) -> ()  [unwired: 2 in, 2 out]
      }
      event "Listbox": Double Click {
        n198 = event-data() -> ("PlatMods.Shift"=w313:bool, "Row"=w315:i32)  [unwired: 1 in]
        n199 = case shown="True" w313 {
          tunnel: w315 -> [w319 _]
          tunnel: 1 -> [w318 _]
          frame False {
            n200 = property on="Listbox" class="LstBox (strict)"() -> ("Item Symbols"=w317:i32[])  [unwired: 2 in, 2 out]
            n201 = Replace Array Subset(array=w317, new element=w318, index=w319) -> (w316:i32[])
            n202 = property on="Listbox" class="LstBox (strict)"("Item Symbols"=w316) -> ()  [unwired: 2 in, 2 out]
          }
          frame True {
            w320 = 0 ("Top Row")
            n203 = property on="Listbox" class="LstBox (strict)"() -> ("Number of Rows"=w322:u32)  [unwired: 2 in, 2 out]
            n204 = Initialize Array(0, w322) -> (w321:i32[])
            n205 = property on="Listbox" class="LstBox (strict)"("Top Row"=w320, "Value"=w320, "Item Symbols"=w321) -> ()  [unwired: 2 in, 2 out]
          }
        }
      }
      event "Listbox": Key Down {
        n206 = event-data() -> ("VKey"=w326:T14)  [unwired: 1 in]
        n207 = case shown="\"Left\", \"Right\"" w326 {
          selector: w326 -> [w331 _]
          tunnel: eventvkey."Left" ("VKey") -> [w329 _]
          frame "Left", "Right" {
            n208 = Equal?(x=w329, y=w331) -> (x = y?=w330:bool)
            n209 = Select(t=0, s=w330, f=1) -> (s? t:f=w332:i32)
            n210 = property on="Listbox" class="LstBox (strict)"() -> ("Item Symbols"=w335:i32[])  [unwired: 2 in, 2 out]
            n211 = Replace Array Subset(array=w335, new element=w332, index="Listbox") -> (w334:i32[])
            n212 = property on="Listbox" class="LstBox (strict)"("Item Symbols"=w334) -> ()  [unwired: 2 in, 2 out]
          }
          frame Default {
          }
        }
      }
      event "DB Camera Config": Value Change {
        n213 = event-data() -> ("NewVal"=w339:bool)  [unwired: 1 in]
        n214 = case shown="False" w339 {
          tunnel: w338 -> [w348 _]
          tunnel: [w341 w359] -> w337
          tunnel: w336 -> [w340 w359]
          frame False {
            w355 = "Camera"
            w358 = FALSE ("Visible")
            n215 = local read "Camera Settings"() -> (w347:T2)
            n216 = Index Array(array=w348) -> (element=w351:cluster{string[]})  [unwired: 1 in]
            n217 = Unbundle(w347) -> ("Frame Rate"=w346:i32, "Compression"=w345:i32, "Size"=w349:u16)
            n218 = Unbundle(w351) -> (w350:string[])
            n219 = Index Array(array=w350, index=w349) -> (element=w344:string)
            n220 = call-poly <vilib>:"Write Key.vi"("section"=w355, "value"=w344, "key"="Size", "refnum"=w340) -> ("refnum out"=w357:T13)  [unwired: 2 in, 5 out]
            n221 = call-poly <vilib>:"Write Key.vi"("section"=w355, "value"=w346, "key"="FrameRate", "refnum"=w357) -> ("refnum out"=w356:T13)  [unwired: 1 in, 6 out]
            n222 = property on="Camera Settings" class="Clust (strict)"("Visible"=w358) -> ()  [unwired: 2 in, 2 out]
            n223 = local write "DB Camera Config"(w358) -> ()
            n224 = call-poly <vilib>:"Write Key.vi"("section"=w355, "value"=w345, "key"="Compression", "refnum"=w356) -> ("refnum out"=w342:T13)  [unwired: 1 in, 6 out]
            n225 = call <vilib>:"Close Config Data.vi"("refnum"=w342) -> ("file path"=w343:path)  [unwired: 2 in, 8 out]
            n226 = call <vilib>:"Open Config Data.vi"("configuration file path"=w343) -> ("refnum"=w341:T13)  [unwired: 8 in, 2 out]
          }
          frame True {
            n227 = property on="Camera Settings" class="Clust (strict)"("Visible"=TRUE) -> ()  [unwired: 2 in, 2 out]
          }
        }
      }
      event "Camera Settings": Value Change {
        n228 = event-data() -> ("NewVal"=w372:T2)  [unwired: 1 in]
        n229 = Index Array(array=w368) -> (element=w367:cluster{string[]})  [unwired: 1 in]
        n230 = Unbundle(w372) -> ("Frame Rate"=w363:i32, "Compression"=w362:i32, "Size"=w365:u16)
        n231 = Unbundle(w367) -> (w366:string[])
        n232 = Index Array(array=w366, index=w365) -> (element=w364:string)
        n233 = Format Into String(format string="%s   %dfps   %d%%", w364, w363, w362) -> (resulting string=w369:string)  [unwired: 2 in, 1 out]
        n234 = Build Array(w369) -> (w370:string[])
        n235 = property on="DB Camera Config" class="Bool (strict)"("Strings [4]"=w370) -> ()  [unwired: 2 in, 2 out]
      }
      event "Motor.Enable": Value Change {
        n236 = event-data() -> ("NewVal"=w378:bool)  [unwired: 1 in]
        n237 = Unbundle("Motor") -> ("Value"=w377:dbl)  [unwired: 1 out]
        n238 = Select(t=w377, s=w378, f=0.0) -> (s? t:f=w375:dbl)
        n239 = call <vilib>:"NT Write Number.vi"("Numeric"=w375, "Name"=w374) -> ()  [unwired: 9 in, 1 out]
      }
      event "Test Slider": Value Change {
        n240 = event-data() -> ("NewVal"=w381:dbl)  [unwired: 1 in]
        n241 = call <vilib>:"NT Write Number.vi"("Numeric"=w381, "Name"=w382) -> ()  [unwired: 9 in, 1 out]
      }
      event "On/Off": Value Change {
        n242 = event-data() -> ("NewVal"=w386:bool)  [unwired: 1 in]
        n243 = Boolean To (0,1)(Boolean=w386) -> (0, 1=w385:i16)
        n244 = call <vilib>:"NT Write Number.vi"("Numeric"=w385, "Name"=w384) -> ()  [unwired: 9 in, 1 out]
      }
      event "Rev/Fwd": Value Change {
        n245 = event-data() -> ("NewVal.Forward"=w394:bool, "NewVal.Reverse"=w393:bool)  [unwired: 1 in]
        n246 = Boolean To (0,1)(Boolean=w394) -> (0, 1=w390:i16)
        n247 = Boolean To (0,1)(Boolean=w393) -> (0, 1=w392:i16)
        n248 = Negate(x=w392) -> (-x=w391:i16)
        n249 = Add(x=w390, y=w391) -> (x+y=w389:i16)
        n250 = call <vilib>:"NT Write Number.vi"("Numeric"=w389, "Name"=w388) -> ()  [unwired: 9 in, 1 out]
      }
      event "Test Ring": Value Change {
        n251 = event-data() -> ("NewVal"=w398:u16)  [unwired: 1 in]
        n252 = property on="Test Ring" class="Ring (strict)"() -> ("Strings []"=w399:string[])  [unwired: 2 in, 2 out]
        n253 = Index Array(array=w399, index=w398) -> (element=w397:string)
        n254 = call <vilib>:"NT Write String.vi"("String"=w397, "Name"=w396) -> ()  [unwired: 9 in, 1 out]
      }
      event "Rec Mode": Value Change {
        # "Update globals for recording mode and path to read log from.\nClear when logging and let NetworkTables set path for vision to\nuse."
        n255 = event-data() -> ("NewVal"=w409:enum32{"Stop", "Record", "Playback"})  [unwired: 1 in]
        n256 = global write "WPI_DashboardLogging Global.vi" "Logging Filename"(path "") -> ()
        n257 = case shown="\"Stop\", \"Record\"" w409 {
          tunnel: w408 -> [_ w411 w419]
          tunnel: [_ _ w418] -> w405
          tunnel: [_ _ w417] -> _
          tunnel: w403 -> [_ _ w415]
          tunnel: cluster{i32, i32} {-250, 170} -> [_ _ w414]
          tunnel: [_ _ T15 {"Image Size"=TRUE, "Image Type"=TRUE, "Pixel Value"=TRUE, "ROI Information"=TRUE, "Zoom Factor"=FALSE} ("Image Information Shown:All Elements")] -> w401
          tunnel: [_ _ TRUE ("Zoom Factor")] -> w400
          frame Default {
          }
          frame "Stop", "Record" {
            # "Place Window too"
            n258 = invoke class="VI" method="FP.Close"(reference=w411) -> (reference out=w410:refnum<vi>)  [unwired: 2 in, 2 out]
            n259 = invoke class="VI" method="Abort VI"(reference=w410) -> ()  [unwired: 2 in, 3 out]
          }
          frame "Playback" {
            n260 = call "Open Playback Panel.vi"("Offset"=w414, "DB VI Ref"=w415, "Playback in"=w419) -> ("Playback out"=w416:refnum<vi>)  [unwired: 8 in]
            n261 = register-events(w416) -> (reference out=w418:refnum<event-registration>, error out=w417:errorcluster)  [unwired: 2 in]
          }
        }
        n262 = global write "WPI_DashboardLogging Global.vi" "Recording"(w409) -> ()
        n263 = property on="Camera Image" class="ImageControl"("Image Information Shown"=w401, "Image Information Visible"=w400) -> ()  [unwired: 2 in, 2 out]
        n264 = call <vilib>:"WPI_DashboardNT Log FieldName Cache.vi"("Operation"=enum16{"Lookup/Add", "Index", "Clear"}."Clear") -> ()  [unwired: 8 in, 3 out]
      }
      event Panel Close {
        w420 = enum32{"Stop", "Record", "Playback"}."Stop" ("Rec Mode")
        n265 = event-data() -> ()  [unwired: 1 in, 4 out]
        n266 = local write "Rec Mode"(w420) -> ()
        n267 = global write "WPI_DashboardLogging Global.vi" "Recording"(w420) -> ()
      }
      event Panel Close {
        # "Abort playback window and ourself"
        n268 = event-data() -> ()  [unwired: 1 in, 4 out]
        n269 = invoke class="VI" method="FP.Close"(reference=w425) -> (reference out=w424:refnum<vi>)  [unwired: 2 in, 2 out]
        n270 = invoke class="VI" method="Abort VI"(reference=w424) -> (error out=w423:errorcluster)  [unwired: 2 in, 2 out]
        n271 = invoke class="VI" method="Abort VI"(error in=w423) -> ()  [unwired: 2 in, 3 out]
      }
    }
  }
  n272 = property on="On/Off" class="Bool (strict)"("Visible"=w24) -> ()  [unwired: 2 in, 2 out]
  n273 = property on="Motor" class="Clust (strict)"("Visible"=w24) -> ()  [unwired: 2 in, 2 out]
  n274 = property on="Progress" class="Clust (strict)"("Visible"=w24) -> ()  [unwired: 2 in, 2 out]
  n275 = property on="Test Ring" class="Ring (strict)"("Visible"=w24) -> ()  [unwired: 2 in, 2 out]
  n276 = property on="Rev/Fwd" class="Clust (strict)"("Visible"=w24) -> ()  [unwired: 2 in, 2 out]
  n277 = property on="Camera Settings" class="Clust (strict)"("Visible"=w24) -> ()  [unwired: 2 in, 2 out]
  n278 = local write "DB Camera Config"(w24) -> ()
  n279 = global write "WPI_DashboardLogging Global.vi" "Recording"(w7) -> ()
  n280 = local write "Rec Mode"(w7) -> ()
